vi "Queues.vi"() -> ()   [LabVIEW 2020]
panel:
  out "In A and B":string[](array[string])
  out "In A not B":string[](array[string])
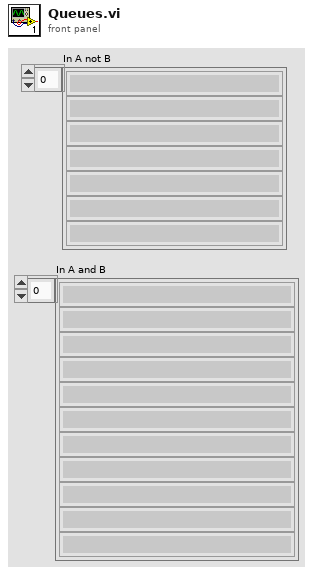
[diagram p1: front panel]
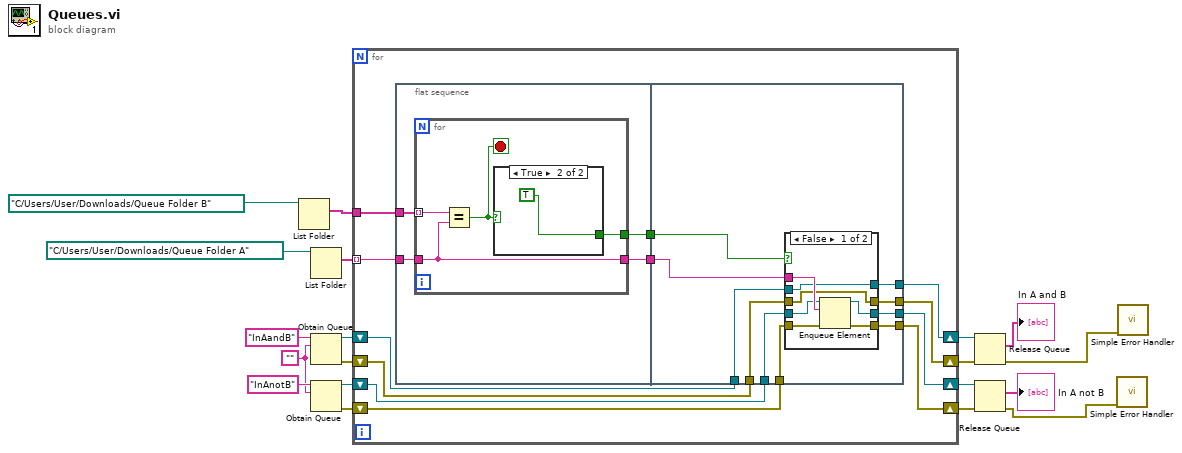
[diagram p0: block diagram]
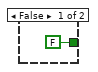
[diagram p2: hidden frame]
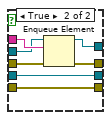
[diagram p3: hidden frame]
diagram:
  w15 = ""
  n1 = List Folder(path=path "C:/Users/User/Downloads/Queue Folder B") -> (filenames=w13:string[])  [unwired: 3 in, 3 out]
  n2 = List Folder(path=path "C:/Users/User/Downloads/Queue Folder A") -> (filenames=w14:string[])  [unwired: 3 in, 3 out]
  n3 = Obtain Queue(name (unnamed)="InAandB", element data type=w15) -> (queue out=w11:refnum<queue>, error out=w6:errorcluster)  [unwired: 3 in, 1 out]
  n4 = Obtain Queue(name (unnamed)="InAnotB", element data type=w15) -> (queue out=w12:refnum<queue>, error out=w5:errorcluster)  [unwired: 3 in, 1 out]
  n5 = for {
    tunnel: w14 -> [w31] mode=indexing
    tunnel: w13 -> [w30]
    shift-right: [w26] -> w10
    shift-left: w11 -> [w28]
    shift-right: [w25] -> w9
    shift-left: w12 -> [w27]
    shift-right: [w21] -> w4
    shift-left: w6 -> [w22]
    shift-right: [w23] -> w3
    shift-left: w5 -> [w24]
    n6 = flat-sequence {
      tunnel: w31 -> [w35]
      tunnel: w30 -> [w34]
      tunnel: [w33] -> w29
      tunnel: [w32] -> w20
      tunnel: w29 -> [w51]
      tunnel: w28 -> [w50]
      tunnel: w27 -> [w49]
      tunnel: [w48] -> w26
      tunnel: [w47] -> w25
      tunnel: w24 -> [w46]
      tunnel: [w45] -> w23
      tunnel: w22 -> [w44]
      tunnel: [w43] -> w21
      tunnel: w20 -> [w42]
      frame #0 {
        n7 = for {
          tunnel: w35 -> [w37]
          tunnel: w34 -> [w38] mode=indexing
          tunnel: [w37] -> w33
          tunnel: [w36] -> w32
          stop <- w39 stop-if-true
          n8 = Equal?(x=w38, y=w37) -> (x = y?=w39:bool)
          n9 = case shown="True" w39 {
            tunnel: [FALSE ("isinb") TRUE ("isinb")] -> w36
            frame False {
            }
            frame True {
            }
          }
        }
      }
      frame #1 {
        n10 = case shown="False" w42 {
          tunnel: w51 -> [w58 w65]
          tunnel: w50 -> [w56 w64]
          tunnel: w49 -> [w57 w62]
          tunnel: [w56 w63] -> w48
          tunnel: [w55 w62] -> w47
          tunnel: w46 -> [w54 w59]
          tunnel: [w53 w59] -> w45
          tunnel: w44 -> [w52 w61]
          tunnel: [w52 w60] -> w43
          frame False {
            n11 = Enqueue Element(queue=w57, element=w58, error in (no error)=w54) -> (queue out=w55:refnum<queue>, error out=w53:errorcluster)  [unwired: 1 in, 1 out]
          }
          frame True {
            n12 = Enqueue Element(queue=w64, element=w65, error in (no error)=w61) -> (queue out=w63:refnum<queue>, error out=w60:errorcluster)  [unwired: 1 in, 1 out]
          }
        }
      }
    }
  }
  n13 = Release Queue(queue=w10, error in (no error)=w4) -> (remaining elements=→"In A and B":string[], error out=w1:errorcluster)  [unwired: 1 in, 1 out]
  n14 = Release Queue(queue=w9, error in (no error)=w3) -> (remaining elements=→"In A not B":string[], error out=w2:errorcluster)  [unwired: 1 in, 1 out]
  n15 = call <vilib>:"Simple Error Handler.vi"("error in (no error)"=w2) -> ()  [unwired: 4 in, 5 out]
  n16 = call <vilib>:"Simple Error Handler.vi"("error in (no error)"=w1) -> ()  [unwired: 4 in, 5 out]
